vi "TDT Stream Test.vi"() -> ()   [LabVIEW 2020]
uses:
  Typedefs/TDT-Output source.ctl
  Typedefs/TDT-Device ID.ctl
  TDT-Signal Bank Action.ctl
  <vilib>/Analysis/NI_AALBase.lvlib
panel:
  out "Graph":dbl[][](graph)
  in  "Frame Size (ms)":dbl=500.0
  in  "AI Sampling Rate (Hz)":dbl=25000.0
  in  "AO Sampling Rate (Hz)":dbl=100000.0
  in  "stop":bool
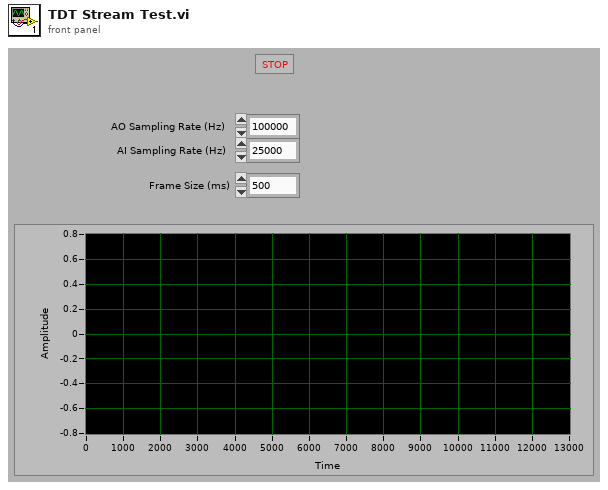
[diagram p1: front panel]
types:
  T1 = typedef "TDT-Signal Bank Action.ctl" = enum16{"Init", "Write", "Read", "Rewrite", "Reset", "Recycle", "Ramp up", "Ramp down", "Zero"}
  T2 = typedef "TDT-Output source.ctl" = cluster{"Device":T3, "Num":i32}
  T3 = typedef "TDT-Device ID.ctl" = enum16{"None", "PA5", "RP2", "RL2", "RA16", "RV8", "RX5", "RX6", "RX7", "RX8", "RZ2", "RZ5", "RZ6"}
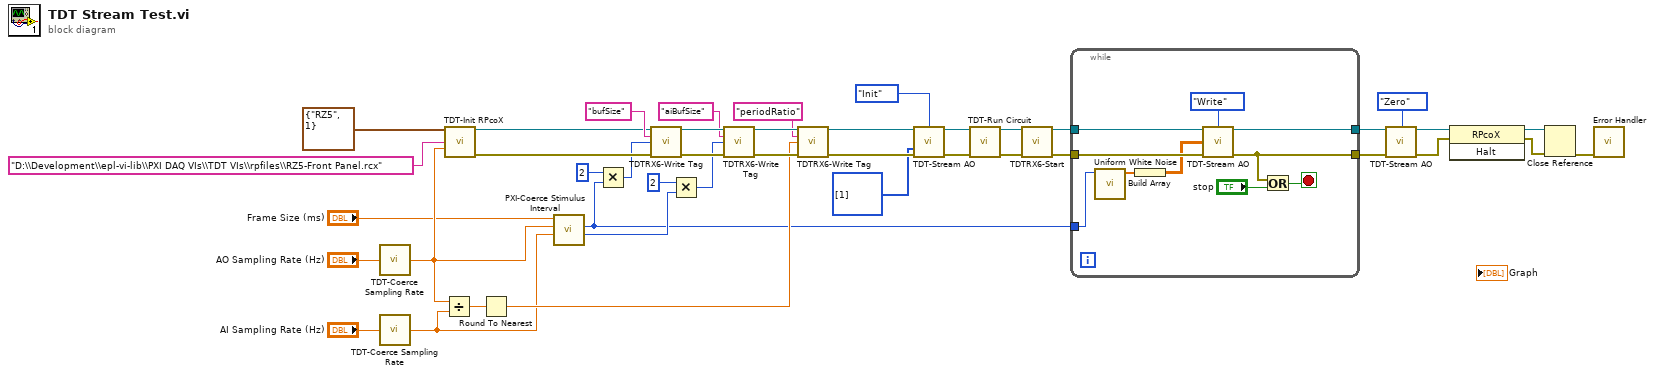
[diagram p0: block diagram]
diagram:
  n1 = call "TDT-Coerce Sampling Rate.vi"("Fs (Hz)"="AO Sampling Rate (Hz)") -> ("Coerced"=w26:dbl)
  n2 = call "TDT-Coerce Sampling Rate.vi"("Fs (Hz)"="AI Sampling Rate (Hz)") -> ("Coerced"=w23:dbl)
  n3 = Divide(x=w26, y=w23) -> (x/y=w31:dbl)
  n4 = call "TDT-Init RPcoX.vi"("Output"=T2 {"Device"=enum."RZ5", "Num"=1}, "RPfilename"="D:\\Development\\epl-vi-lib\\PXI DAQ VIs\\TDT VIs\\rpfiles\\RZ5-Front Panel.rcx", "Sampling rate (Hz)"=w26) -> ("RPcoX"=w22:refnum<k7>, "error out"=w21:errorcluster)  [unwired: 11 in]
  n5 = Round To Nearest(number=w31) -> (nearest integer value=w30:dbl)
  n6 = call "PXI-Coerce Stimulus Interval.vi"("AI sampling rate (Hz)"=w23, "AO sampling rate (Hz)"=w26, "Stimulus interval (ms)"="Frame Size (ms)") -> ("AI npts"=w28:i32, "AO npts"=w5:i32)  [unwired: 5 in, 2 out]
  n7 = Multiply(x=2, y=w5) -> (x*y=w19:i32)
  n8 = call "TDTRX6-Write Tag.vi"("RPcox"=w22, "Name"="bufSize", "Value"=w19, "error in"=w21) -> ("RPcox Out"=w36:refnum<k7>, "error out"=w37:errorcluster)  [unwired: 10 in]
  n9 = Multiply(x=2, y=w28) -> (x*y=w29:i32)
  n10 = call "TDTRX6-Write Tag.vi"("RPcox"=w36, "Name"="aiBufSize", "Value"=w29, "error in"=w37) -> ("RPcox Out"=w33:refnum<k7>, "error out"=w34:errorcluster)  [unwired: 10 in]
  n11 = call "TDTRX6-Write Tag.vi"("RPcox"=w33, "Name"="periodRatio", "Value"=w30, "error in"=w34) -> ("RPcox Out"=w14:refnum<k7>, "error out"=w17:errorcluster)  [unwired: 10 in]
  n12 = call "TDT-Stream AO.vi"("RPcox"=w14, "Action"=TDT-Signal_Bank_Action."Init", "Chans"=i32[] [1], "error in (no error)"=w17) -> ("RPcox thru"=w13:refnum<k7>, "error out"=w15:errorcluster)  [unwired: 10 in]
  n13 = call "TDT-Run Circuit.vi"("RPcoX"=w13, "error in (no error)"=w15) -> ("RPcoX out"=w2:refnum<k7>, "error out"=w4:errorcluster)  [unwired: 12 in]
  n14 = call "TDTRX6-Start.vi"("error in (no error)"=w4) -> ("error out"=w3:errorcluster)  [unwired: 6 in]
  n15 = while {
    tunnel: w3 -> [w50]
    tunnel: [w45] -> w10
    tunnel: w2 -> [w44]
    tunnel: [w43] -> w12
    tunnel: w5 -> [w42]
    stop <- w46 stop-if-true
    n16 = call <vilib>:"Uniform White Noise.vi"("samples"=w42) -> ("uniform white noise"=w51:dbl[])  [unwired: 9 in, 1 out]
    n17 = Build Array(w51) -> (w49:dbl[][])
    n18 = call "TDT-Stream AO.vi"("RPcox"=w44, "Action"=TDT-Signal_Bank_Action."Write", "Output array"=w49, "error in (no error)"=w50) -> ("RPcox thru"=w43:refnum<k7>, "error out"=w45:errorcluster)  [unwired: 10 in]
    n19 = Or(x=w45, y="stop") -> (x .or. y?=w46:bool)
  }
  n20 = call "TDT-Stream AO.vi"("RPcox"=w12, "Action"=TDT-Signal_Bank_Action."Zero", "error in (no error)"=w10) -> ("RPcox thru"=w1:refnum<k7>, "error out"=w9:errorcluster)  [unwired: 11 in]
  n21 = invoke class="RPcoX" method="Halt"(reference=w1, error in=w9) -> (reference out=w8:refnum<k7>, error out=w7:errorcluster)  [unwired: 1 in, 1 out]
  n22 = Close Reference(reference=w8, error in (no error)=w7) -> (error out=w6:errorcluster)
  n23 = call "Error Handler.vi"("error in (no error)"=w6) -> ()  [unwired: 12 in, 3 out]
